vi "nanocal -- nuclear schottky fit V8.vi"() -> ()   [LabVIEW 2021] (continued)
  out "color data":cluster{"Array":dbl[], "Array":dbl[]}[](array[cluster])=[{"Array"=[0.12, 0.148, 0.179, 0.197, 0.249, 0.3, 0.36, 0.43, 0.512, 0.61, 0.81, 1.1, 1.8, 3.0, 5.7], "Array"=[0.375235391174, 0.267189614091, 0.199306617611, 0.169435500052, 0.10023219366, 0.068889386962, 0.050855621628, 0.038379394547, 0.030757711173, 0.024472356387, 0.019125590894, 0.016340595254, 0.01263439258, 0.019026086981, 0.019858524497]}, {"Array"=[0.12, 0.148, 0.179, 0.197, 0.249, 0.3, 0.36, 0.43, 0.512, 0.61, 0.81, 1.1, 1.8, 3.0, 5.7], "Array"=[0.100390183494, 0.086925369127, 0.070107577087, 0.06552222252, 0.0499817149, 0.042189760597, 0.035114064267, 0.030049345911, 0.024931554661, 0.022407083343, 0.016432131318, 0.01691523202, 0.012311180561, 0.018297259133, 0.012821278093]}, {"Array"=[0.12, 0.148, 0.179, 0.197, 0.249, 0.3, 0.36, 0.43, 0.512, 0.61, 0.81, 1.1, 1.8, 3.0, 5.7], "Array"=[0.059883674441, 0.044416499058, 0.034354681127, 0.031885966152, 0.026964705596, 0.023837806105, 0.021745076003, 0.020197203084, 0.019059366283, 0.017600386438, 0.016139955363, 0.015114072822, 0.011880374999, 0.007367031681, 0.004631070276]}, {"Array"=[0.12, 0.148, 0.179, 0.197, 0.249, 0.3, 0.36, 0.43, 0.512, 0.61, 0.81, 1.1, 1.8, 3.0, 5.7], "Array"=[0.583268417564, 0.254096954422, 0.115326183519, 0.085736532349, 0.034498560244, 0.017176281362, 0.009940720882, 0.005279271749, 0.002804912424, 0.001730254025, 0.000695948251, 0.000265648688, 6.6834392e-05, 1.2328467e-05, 1.621029e-06]}, {"Array"=[0.12, 0.148, 0.179, 0.197, 0.249, 0.3, 0.36, 0.43, 0.512, 0.61, 0.81, 1.1, 1.8, 3.0, 5.7], "Array"=[0.00101538821, 0.000963914391, 0.001029913549, 0.00108551185, 0.001422553924, 0.001657645209, 0.002035754152, 0.002296433055, 0.00240095569, 0.003444856237, 0.003787605771, 0.003610389555, 0.00409358538, 0.005085235141, 0.003887972994]}, {"Array"=[0.12, 0.148, 0.179, 0.197, 0.249, 0.3, 0.36, 0.43, 0.512, 0.61, 0.81, 1.1, 1.8, 3.0, 5.7], "Array"=[4.51e-10, 6.59e-10, 9.06e-10, 1.071e-09, 1.37e-09, 1.746e-09, 2.124e-09, 2.676e-09, 3.344e-09, 3.989e-09, 5.582e-09, 7.797e-09, 1.3452e-08, 2.3922e-08, 5.8873e-08]}, {"Array"=[0.12, 0.148, 0.179, 0.197, 0.249, 0.3, 0.36, 0.43, 0.512, 0.61, 0.81, 1.1, 1.8, 3.0, 5.7], "Array"=[0.000375271363, 0.000162673595, 8.029081e-05, 5.7538627e-05, 9.1233173e-05, 7.1502532e-05, 5.116404e-05, 5.9898317e-05, 8.8127283e-05, 8.7154359e-05, 0.000129667374, 0.000367130935, 0.000860954265, 0.473735460179, 6.096146916988]}, {"Array"=[0.12, 0.148, 0.179, 0.197, 0.249, 0.3, 0.36, 0.43, 0.512, 0.61, 0.81, 1.1, 1.8, 3.0, 5.7], "Array"=[0.000128650872, 3.6959811e-05, 1.3361577e-05, 8.322484e-06, 9.463067e-06, 5.082442e-06, 2.904884e-06, 2.370734e-06, 2.53316e-06, 1.846195e-06, 1.793381e-06, 1.790268e-06, 1.598192e-06, 0.000298320672, 0.000788360465]}, {"Array"=[0.12, 0.148, 0.179, 0.197, 0.249, 0.3, 0.36, 0.43, 0.512, 0.61, 0.81, 1.1, 1.8, 3.0, 5.7], "Array"=[0.00159846382, 0.000362772077, 0.000100930245, 5.7382706e-05, 4.5871847e-05, 2.0526312e-05, 9.775078e-06, 6.802565e-06, 6.068263e-06, 3.983538e-06, 2.982571e-06, 3.209434e-06, 2.482039e-06, 0.226260580227, 2.944305334628]}, {"Array"=[0.12, 0.148, 0.179, 0.197, 0.249, 0.3, 0.36, 0.43, 0.512, 0.61, 0.81, 1.1, 1.8, 3.0, 5.7], "Array"=[0.003738128067, 0.00187141679, 0.001145251526, 0.000878154381, 0.00182533099, 0.001694784024, 0.001457081108, 0.001993331815, 0.003534768852, 0.003889589636, 0.007891086787, 0.021704161954, 0.06993271366, 0.0, 0.0]}, {"Array"=[0.12, 0.148, 0.179, 0.197, 0.249, 0.3, 0.36, 0.43, 0.512, 0.61, 0.81, 1.1, 1.8, 3.0, 5.7], "Array"=[0.002148346326, 0.000832118957, 0.000388930305, 0.000261007731, 0.000350942719, 0.000213209307, 0.000133588143, 0.000117379325, 0.00013290891, 0.000104895132, 0.000111114402, 0.000118450384, 0.000134523688, 0.0, 0.0]}, {"Array"=[0.12, 0.148, 0.179, 0.197, 0.249, 0.3, 0.36, 0.43, 0.512, 0.61, 0.81, 1.1, 1.8, 3.0, 5.7], "Array"=[0.002740528669, 0.00142769156, 0.000875171988, 0.000669291195, 0.001329674256, 0.00119503816, 0.000983336979, 0.001288542279, 0.002163441144, 0.002302284973, 0.004285622428, 0.012081499151, 0.037137152263, 0.0, 0.0]}, {"Array"=[0.12, 0.148, 0.179, 0.197, 0.249, 0.3, 0.36, 0.43, 0.512, 0.61, 0.81, 1.1, 1.8, 3.0, 5.7], "Array"=[0.004856405038, 0.00339935422, 0.002396778835, 0.002148162128, 0.001574610259, 0.001314390211, 0.001126696289, 0.000994558397, 0.000873567124, 0.000814716505, 0.00067871105, 0.000664500257, 0.000525383024, 0.0, 0.0]}, {"Array"=[0.12, 0.148, 0.179, 0.197, 0.249, 0.3, 0.36, 0.43, 0.512, 0.61, 0.81, 1.1, 1.8, 3.0, 5.7], "Array"=[0.000120937865, 6.5769536e-05, 3.6147224e-05, 2.8270387e-05, 1.5357324e-05, 8.848315e-06, 6.319561e-06, 4.045439e-06, 2.751674e-06, 1.970451e-06, 1.210723e-06, 3.99152e-07, 1.29432e-07, 0.0, 0.0]}, {"Array"=[0.12, 0.148, 0.179, 0.197, 0.249, 0.3, 0.36, 0.43, 0.512, 0.61, 0.81, 1.1, 1.8, 3.0, 5.7], "Array"=[0.036262763887, 0.013360978569, 0.005461206603, 0.003934877132, 0.001506729222, 0.000735278812, 0.000424808302, 0.000225535524, 0.000120705086, 7.4828897e-05, 3.0773e-05, 1.1616244e-05, 2.96677e-06, 0.0, 0.0]}, {"Array"=[0.12, 0.148, 0.179, 0.197, 0.249, 0.3, 0.36, 0.43, 0.512, 0.61, 0.81, 1.1, 1.8, 3.0, 5.7], "Array"=[0.04837529795, 0.039106583663, 0.034187158287, 0.032785245148, 0.03150372616, 0.031154246719, 0.032086752475, 0.033097505686, 0.03503861415, 0.036359774839, 0.041303896436, 0.039284134925, 0.042675275628, 0.0, 0.0]}, {"Array"=[0.12, 0.148, 0.179, 0.197, 0.249, 0.3, 0.36, 0.43, 0.512, 0.61, 0.81, 1.1, 1.8, 3.0, 5.7], "Array"=[0.0020195465, 0.001480745607, 0.001052177546, 0.000886609066, 0.000569534267, 0.000371188322, 0.00029062032, 0.000200297015, 0.000144373831, 0.000111954983, 7.5013998e-05, 2.6409322e-05, 1.0894575e-05, 0.0, 0.0]}, {"Array"=[0.12, 0.148, 0.179, 0.197, 0.249, 0.3, 0.36, 0.43, 0.512, 0.61, 0.81, 1.1, 1.8, 3.0, 5.7], "Array"=[0.062171656813, 0.05258220666, 0.047354437967, 0.045894988103, 0.043675133431, 0.042807799707, 0.042734154502, 0.042720953668, 0.043033459724, 0.043247347257, 0.044217367932, 0.043727840988, 0.044389870063, 0.0, 0.0]}, {"Array"=[0.12, 0.148, 0.179, 0.197, 0.249, 0.3, 0.36, 0.43, 0.512, 0.61, 0.81, 1.1, 1.8, 3.0, 5.7], "Array"=[0.0, 0.0, 0.0, 0.0, 0.0, 0.0, 0.0, 0.0, 0.0, 0.0, 0.0, 0.0, 0.0, -126530.61224489775, -53061.22448979574]}, {"Array"=[0.12, 0.148, 0.179, 0.197, 0.249, 0.3, 0.36, 0.43, 0.512, 0.61, 0.81, 1.1, 1.8, 3.0, 5.7], "Array"=[0.0, 0.0, 0.0, 0.0, 0.0, 0.0, 0.0, 0.0, 0.0, 0.0, 0.0, 0.0, 0.0, 0.0, 0.0]}, {"Array"=[0.12, 0.148, 0.179, 0.197, 0.249, 0.3, 0.36, 0.43, 0.512, 0.61, 0.81, 1.1, 1.8, 3.0, 5.7], "Array"=[0.0, 0.0, 0.0, 0.0, 0.0, 0.0, 0.0, 0.0, 0.0, 0.0, 0.0, 0.0, 0.0, 0.0, 0.0]}]
  out "R(ω) fit out":cdb[](array[numeric])
  in  "parameter map":map{T1, dbl}(c390)={enum."ζ"=0.068889386962, enum."τ1"=0.042189760597, enum."τS"=0.023837806105, enum."τN"=0.017176281362, enum."τC"=0.001657645209, enum."κ0"=1.746e-09}
  out "filesnames lookup":map{i32, string}(c390)={0="IDS0158_210310_RAW_cal__sam_", 1="IDS0183_210310_RAW_cal__sam_", 2="IDS0311_210901_RAW_cal__sam_", 3="IDS0359_210907_RAW_cal__sam_", 4="IDS0412_220525_RAW_cal__sam_", 5="IDS0431_220527_RAW_cal__sam_", 6="IDS0442_220528_RAW_cal__sam_", 7="IDS0464_220530_RAW_cal__sam_", 8="IDS0486_220602_RAW_cal__sam_", 9="IDS0495_220602_RAW_cal__sam_", 10="IDS0510_220603_RAW_cal__sam_", 11="IDS0526_220605_RAW_cal__sam_", 12="IDS0544_220606_RAW_cal__sam_", 13="IDS0561_220607_RAW_cal__sam_", 14="IDS0581_220608_RAW_cal__sam_", 15="IDS0598_220609_RAW_cal__sam_", 16="IDS0627_220611_RAW_cal__sam_", 17="IDS0643_220612_RAW_cal__sam_", 18="IDS0336_210904_RAW_cal__sam_", 19="IDS0346_210904_RAW_cal__sam_", 20="IDS0378_210909_RAW_cal__sam_", 21="IDS0300_210427_RAW_cal__sam_", 22="IDS0184_210310_RAW_cal__sam_", 23="IDS0210_210310_RAW_cal__sam_", 24="IDS0379_210909_RAW_cal__sam_", 25="IDS0159_210310_RAW_cal__sam_", 26="IDS0360_210907_RAW_cal__sam_", 27="IDS0411_220525_RAW_cal__sam_", 28="IDS0427_220526_RAW_cal__sam_", 29="IDS0443_220528_RAW_cal__sam_", 30="IDS0463_220530_RAW_cal__sam_", 31="IDS0487_220602_RAW_cal__sam_", 32="IDS0496_220602_RAW_cal__sam_", 33="IDS0509_220603_RAW_cal__sam_", 34="IDS0525_220605_RAW_cal__sam_", 35="IDS0543_220606_RAW_cal__sam_", 36="IDS0560_220607_RAW_cal__sam_", 37="IDS0580_220608_RAW_cal__sam_", 38="IDS0597_220608_RAW_cal__sam_", 39="IDS0626_220611_RAW_cal__sam_", 40="IDS0642_220612_RAW_cal__sam_", 41="IDS0310_210901_RAW_cal__sam_", 42="IDS0337_210904_RAW_cal__sam_", 43="IDS0347_210906_RAW_cal__sam_", 44="IDS0305_210831_RAW_cal__sam_", 45="IDS0361_210908_RAW_cal__sam_", 46="IDS0380_210909_RAW_cal__sam_", 47="IDS0304_210831_RAW_cal__sam_", 48="IDS0312_210901_RAW_cal__sam_", 49="IDS0338_210904_RAW_cal__sam_", 50="IDS0410_220525_RAW_cal__sam_", 51="IDS0432_220527_RAW_cal__sam_", 52="IDS0444_220528_RAW_cal__sam_", 53="IDS0462_220530_RAW_cal__sam_", 54="IDS0485_220601_RAW_cal__sam_", 55="IDS0497_220603_RAW_cal__sam_", 56="IDS0511_220604_RAW_cal__sam_", 57="IDS0524_220605_RAW_cal__sam_", 58="IDS0542_220606_RAW_cal__sam_", 59="IDS0559_220607_RAW_cal__sam_", 60="IDS0579_220608_RAW_cal__sam_", 61="IDS0596_220608_RAW_cal__sam_", 62="IDS0625_220611_RAW_cal__sam_", 63="IDS0641_220612_RAW_cal__sam_", 64="IDS0348_210906_RAW_cal__sam_", 65="IDS0181_210310_RAW_cal__sam_", 66="IDS0160_210310_RAW_cal__sam_", 67="IDS0424_220526_RAW_cal__sam_", 68="IDS0185_210310_RAW_cal__sam_", 69="IDS0208_210310_RAW_cal__sam_", 70="IDS0209_210310_RAW_cal__sam_", 71="IDS0211_210310_RAW_cal__sam_", 72="IDS0212_210310_RAW_cal__sam_", 73="IDS0213_210310_RAW_cal__sam_", 74="IDS0214_210310_RAW_cal__sam_", 75="IDS0215_210310_RAW_cal__sam_", 76="IDS0216_210310_RAW_cal__sam_", 77="IDS0217_210310_RAW_cal__sam_", 78="IDS0330_210901_RAW_cal__sam_", 79="IDS0331_210901_RAW_cal__sam_", 80="IDS0335_210904_RAW_cal__sam_", 81="IDS0362_210908_RAW_cal__sam_", 82="IDS0377_210909_RAW_cal__sam_", 83="IDS0161_210310_RAW_cal__sam_", 84="IDS0303_210831_RAW_cal__sam_", 85="IDS0313_210901_RAW_cal__sam_", 86="IDS0349_210906_RAW_cal__sam_", 87="IDS0407_220525_RAW_cal__sam_", 88="IDS0441_220527_RAW_cal__sam_", 89="IDS0458_220529_RAW_cal__sam_", 90="IDS0477_220601_RAW_cal__sam_", 91="IDS0493_220602_RAW_cal__sam_", 92="IDS0508_220603_RAW_cal__sam_", 93="IDS0523_220604_RAW_cal__sam_", 94="IDS0540_220605_RAW_cal__sam_", 95="IDS0562_220607_RAW_cal__sam_", 96="IDS0578_220608_RAW_cal__sam_", 97="IDS0595_220608_RAW_cal__sam_", 98="IDS0624_220611_RAW_cal__sam_", 99="IDS0640_220612_RAW_cal__sam_", 100="IDS0186_210310_RAW_cal__sam_", 101="IDS0162_210310_RAW_cal__sam_", 102="IDS0302_210831_RAW_cal__sam_", 103="IDS0363_210908_RAW_cal__sam_", 104="IDS0381_210909_RAW_cal__sam_", 105="IDS0408_220525_RAW_cal__sam_", 106="IDS0425_220526_RAW_cal__sam_", 107="IDS0445_220528_RAW_cal__sam_", 108="IDS0459_220529_RAW_cal__sam_", 109="IDS0478_220601_RAW_cal__sam_", 110="IDS0494_220602_RAW_cal__sam_", 111="IDS0512_220604_RAW_cal__sam_", 112="IDS0527_220605_RAW_cal__sam_", 113="IDS0541_220605_RAW_cal__sam_", 114="IDS0563_220607_RAW_cal__sam_", 115="IDS0582_220608_RAW_cal__sam_", 116="IDS0599_220609_RAW_cal__sam_", 117="IDS0628_220611_RAW_cal__sam_", 118="IDS0644_220612_RAW_cal__sam_", 119="IDS0314_210901_RAW_cal__sam_", 120="IDS0339_210904_RAW_cal__sam_", 121="IDS0350_210906_RAW_cal__sam_", 122="IDS0163_210310_RAW_cal__sam_", 123="IDS0187_210310_RAW_cal__sam_", 124="IDS0301_210831_RAW_cal__sam_", 125="IDS0315_210901_RAW_cal__sam_", 126="IDS0382_210909_RAW_cal__sam_", 127="IDS0409_220525_RAW_cal__sam_", 128="IDS0426_220526_RAW_cal__sam_", 129="IDS0446_220528_RAW_cal__sam_", 130="IDS0460_220529_RAW_cal__sam_", 131="IDS0479_220601_RAW_cal__sam_", 132="IDS0498_220603_RAW_cal__sam_", 133="IDS0513_220604_RAW_cal__sam_", 134="IDS0528_220605_RAW_cal__sam_", 135="IDS0545_220606_RAW_cal__sam_", 136="IDS0564_220607_RAW_cal__sam_", 137="IDS0583_220608_RAW_cal__sam_", 138="IDS0629_220611_RAW_cal__sam_", 139="IDS0645_220612_RAW_cal__sam_", 140="IDS0656_220614_RAW_cal__sam_", 141="IDS0364_210908_RAW_cal__sam_", 142="IDS0340_210904_RAW_cal__sam_", 143="IDS0351_210906_RAW_cal__sam_", 144="IDS0164_210310_RAW_cal__sam_", 145="IDS0188_210310_RAW_cal__sam_", 146="IDS0299_210427_RAW_cal__sam_", 147="IDS0316_210901_RAW_cal__sam_", 148="IDS0341_210904_RAW_cal__sam_", 149="IDS0352_210906_RAW_cal__sam_", 150="IDS0365_210908_RAW_cal__sam_", 151="IDS0383_210910_RAW_cal__sam_", 152="IDS0413_220525_RAW_cal__sam_", 153="IDS0428_220526_RAW_cal__sam_", 154="IDS0447_220528_RAW_cal__sam_", 155="IDS0461_220529_RAW_cal__sam_", 156="IDS0480_220601_RAW_cal__sam_", 157="IDS0499_220603_RAW_cal__sam_", 158="IDS0514_220604_RAW_cal__sam_", 159="IDS0529_220605_RAW_cal__sam_", 160="IDS0546_220606_RAW_cal__sam_", 161="IDS0565_220607_RAW_cal__sam_", 162="IDS0584_220608_RAW_cal__sam_", 163="IDS0601_220609_RAW_cal__sam_", 164="IDS0630_220611_RAW_cal__sam_", 165="IDS0646_220612_RAW_cal__sam_", 166="IDS0429_220526_RAW_cal__sam_", 167="IDS0448_220528_RAW_cal__sam_", 168="IDS0481_220601_RAW_cal__sam_", 169="IDS0500_220603_RAW_cal__sam_", 170="IDS0530_220605_RAW_cal__sam_", 171="IDS0547_220606_RAW_cal__sam_", 172="IDS0566_220607_RAW_cal__sam_", 173="IDS0585_220608_RAW_cal__sam_", 174="IDS0602_220609_RAW_cal__sam_", 175="IDS0631_220611_RAW_cal__sam_", 176="IDS0647_220612_RAW_cal__sam_", 177="IDS0165_210310_RAW_cal__sam_", 178="IDS0189_210310_RAW_cal__sam_", 179="IDS0298_210427_RAW_cal__sam_", 180="IDS0317_210901_RAW_cal__sam_", 181="IDS0366_210908_RAW_cal__sam_", 182="IDS0384_210910_RAW_cal__sam_", 183="IDS0414_220525_RAW_cal__sam_", 184="IDS0465_220530_RAW_cal__sam_", 185="IDS0515_220604_RAW_cal__sam_", 186="IDS0342_210904_RAW_cal__sam_", 187="IDS0353_210906_RAW_cal__sam_", 188="IDS0190_210310_RAW_cal__sam_", 189="IDS0166_210310_RAW_cal__sam_", 190="IDS0430_220526_RAW_cal__sam_", 191="IDS0449_220528_RAW_cal__sam_", 192="IDS0482_220601_RAW_cal__sam_", 193="IDS0501_220603_RAW_cal__sam_", 194="IDS0516_220604_RAW_cal__sam_", 195="IDS0531_220605_RAW_cal__sam_", 196="IDS0548_220606_RAW_cal__sam_", 197="IDS0567_220607_RAW_cal__sam_", 198="IDS0586_220608_RAW_cal__sam_", 199="IDS0603_220609_RAW_cal__sam_", 200="IDS0632_220611_RAW_cal__sam_", 201="IDS0648_220613_RAW_cal__sam_", 202="IDS0297_210427_RAW_cal__sam_", 203="IDS0318_210901_RAW_cal__sam_", 204="IDS0343_210904_RAW_cal__sam_", 205="IDS0354_210906_RAW_cal__sam_", 206="IDS0367_210908_RAW_cal__sam_", 207="IDS0385_210910_RAW_cal__sam_", 208="IDS0415_220525_RAW_cal__sam_", 209="IDS0466_220530_RAW_cal__sam_", 210="IDS0191_210310_RAW_cal__sam_", 211="IDS0167_210310_RAW_cal__sam_", 212="IDS0296_210427_RAW_cal__sam_", 213="IDS0319_210901_RAW_cal__sam_", 214="IDS0344_210904_RAW_cal__sam_", 215="IDS0433_220527_RAW_cal__sam_", 216="IDS0450_220528_RAW_cal__sam_", 217="IDS0467_220530_RAW_cal__sam_", 218="IDS0483_220601_RAW_cal__sam_", 219="IDS0502_220603_RAW_cal__sam_", 220="IDS0517_220604_RAW_cal__sam_", 221="IDS0532_220605_RAW_cal__sam_", 222="IDS0549_220606_RAW_cal__ref_", 223="IDS0568_220607_RAW_cal__sam_", 224="IDS0587_220608_RAW_cal__sam_", 225="IDS0604_220609_RAW_cal__sam_", 226="IDS0618_220610_RAW_cal__sam_", 227="IDS0633_220611_RAW_cal__sam_", 228="IDS0649_220613_RAW_cal__sam_", 229="IDS0368_210908_RAW_cal__sam_", 230="IDS0386_210910_RAW_cal__sam_", 231="IDS0416_220525_RAW_cal__sam_", 232="IDS0220_210310_RAW_cal__sam_", 233="IDS0168_210310_RAW_cal__sam_", 234="IDS0192_210310_RAW_cal__sam_", 235="IDS0434_220527_RAW_cal__sam_", 236="IDS0451_220528_RAW_cal__sam_", 237="IDS0468_220530_RAW_cal__sam_", 238="IDS0484_220601_RAW_cal__sam_", 239="IDS0503_220603_RAW_cal__sam_", 240="IDS0518_220604_RAW_cal__sam_", 241="IDS0533_220605_RAW_cal__sam_", 242="IDS0550_220606_RAW_cal__sam_", 243="IDS0569_220607_RAW_cal__sam_", 244="IDS0588_220608_RAW_cal__sam_", 245="IDS0605_220609_RAW_cal__sam_", 246="IDS0612_220610_RAW_cal__sam_", 247="IDS0634_220612_RAW_cal__sam_", 248="IDS0650_220613_RAW_cal__sam_", 249="IDS0295_210427_RAW_cal__sam_", 250="IDS0320_210901_RAW_cal__sam_", 251="IDS0355_210906_RAW_cal__sam_", 252="IDS0369_210908_RAW_cal__sam_", 253="IDS0387_210910_RAW_cal__sam_", 254="IDS0417_220525_RAW_cal__sam_", 255="IDS0219_210310_RAW_cal__sam_", 256="IDS0193_210310_RAW_cal__sam_", 257="IDS0606_220609_RAW_cal__sam_", 258="IDS0169_210310_RAW_cal__sam_", 259="IDS0418_220525_RAW_cal__sam_", 260="IDS0435_220527_RAW_cal__sam_", 261="IDS0452_220528_RAW_cal__sam_", 262="IDS0469_220530_RAW_cal__sam_", 263="IDS0488_220602_RAW_cal__sam_", 264="IDS0504_220603_RAW_cal__sam_", 265="IDS0519_220604_RAW_cal__sam_", 266="IDS0534_220605_RAW_cal__sam_", 267="IDS0551_220606_RAW_cal__sam_", 268="IDS0570_220607_RAW_cal__sam_", 269="IDS0589_220608_RAW_cal__sam_", 270="IDS0613_220610_RAW_cal__sam_", 271="IDS0619_220610_RAW_cal__sam_", 272="IDS0635_220612_RAW_cal__sam_", 273="IDS0651_220613_RAW_cal__sam_", 274="IDS0294_210427_RAW_cal__sam_", 275="IDS0321_210901_RAW_cal__sam_", 276="IDS0370_210908_RAW_cal__sam_", 277="IDS0388_210910_RAW_cal__sam_", 278="IDS0391_210910_RAW_cal__sam_", 279="IDS0439_220527_RAW_cal__sam_", 280="IDS0395_210910_RAW_cal__sam_", 281="IDS0392_210910_RAW_cal__sam_", 282="IDS0556_220606_RAW_cal__sam_", 283="IDS0389_210910_RAW_cal__sam_", 284="IDS0218_210310_RAW_cal__sam_", 285="IDS0590_220608_RAW_cal__sam_", 286="IDS0607_220609_RAW_cal__sam_", 287="IDS0453_220529_RAW_cal__sam_", 288="IDS0535_220605_RAW_cal__sam_", 289="IDS0170_210310_RAW_cal__sam_", 290="IDS0194_210310_RAW_cal__sam_", 291="IDS0293_210427_RAW_cal__sam_", 292="IDS0322_210901_RAW_cal__sam_", 293="IDS0371_210908_RAW_cal__sam_", 294="IDS0390_210910_RAW_cal__sam_", 295="IDS0419_220525_RAW_cal__sam_", 296="IDS0436_220527_RAW_cal__sam_", 297="IDS0454_220529_RAW_cal__sam_", 298="IDS0470_220530_RAW_cal__sam_", 299="IDS0489_220602_RAW_cal__sam_", 300="IDS0505_220603_RAW_cal__sam_", 301="IDS0520_220604_RAW_cal__sam_", 302="IDS0536_220605_RAW_cal__sam_", 303="IDS0552_220606_RAW_cal__sam_", 304="IDS0571_220607_RAW_cal__sam_", 305="IDS0608_220610_RAW_cal__sam_", 306="IDS0614_220610_RAW_cal__sam_", 307="IDS0620_220610_RAW_cal__sam_", 308="IDS0636_220612_RAW_cal__sam_", 309="IDS0652_220613_RAW_cal__sam_", 310="IDS0420_220525_RAW_cal__sam_", 311="IDS0421_220525_RAW_cal__sam_", 312="IDS0471_220530_RAW_cal__sam_", 313="IDS0553_220606_RAW_cal__sam_", 314="IDS0572_220607_RAW_cal__sam_", 315="IDS0591_220608_RAW_cal__sam_", 316="IDS0195_210310_RAW_cal__sam_", 317="IDS0472_220530_RAW_cal__sam_", 318="IDS0171_210310_RAW_cal__sam_", 319="IDS0306_210831_RAW_cal__sam_", 320="IDS0323_210901_RAW_cal__sam_", 321="IDS0422_220525_RAW_cal__sam_", 322="IDS0437_220527_RAW_cal__sam_", 323="IDS0455_220529_RAW_cal__sam_", 324="IDS0490_220602_RAW_cal__sam_", 325="IDS0506_220603_RAW_cal__sam_", 326="IDS0521_220604_RAW_cal__sam_", 327="IDS0537_220605_RAW_cal__sam_", 328="IDS0554_220606_RAW_cal__sam_", 329="IDS0573_220607_RAW_cal__sam_", 330="IDS0592_220608_RAW_cal__sam_", 331="IDS0609_220610_RAW_cal__sam_", 332="IDS0615_220610_RAW_cal__sam_", 333="IDS0621_220610_RAW_cal__sam_", 334="IDS0637_220612_RAW_cal__sam_", 335="IDS0653_220613_RAW_cal__sam_", 336="IDS0372_210908_RAW_cal__sam_", 337="IDS0393_210910_RAW_cal__sam_", 338="IDS0172_210310_RAW_cal__sam_", 339="IDS0196_210310_RAW_cal__sam_", 340="IDS0324_210901_RAW_cal__sam_", 341="IDS0438_220527_RAW_cal__sam_", 342="IDS0456_220529_RAW_cal__sam_", 343="IDS0473_220531_RAW_cal__sam_", 344="IDS0491_220602_RAW_cal__sam_", 345="IDS0538_220605_RAW_cal__sam_", 346="IDS0555_220606_RAW_cal__sam_", 347="IDS0574_220607_RAW_cal__sam_", 348="IDS0593_220608_RAW_cal__sam_", 349="IDS0610_220610_RAW_cal__sam_", 350="IDS0616_220610_RAW_cal__sam_", 351="IDS0622_220610_RAW_cal__sam_", 352="IDS0638_220612_RAW_cal__sam_", 353="IDS0654_220613_RAW_cal__sam_", 354="IDS0373_210908_RAW_cal__sam_", 355="IDS0394_210910_RAW_cal__sam_"}
  out "constrained filename lookup":map{i32, string}(c390)={0="IDS0183_210310_RAW_cal__ref_", 1="IDS0184_210310_RAW_cal__ref_", 2="IDS0181_210310_RAW_cal__ref_", 3="IDS0185_210310_RAW_cal__ref_", 4="IDS0186_210310_RAW_cal__ref_", 5="IDS0187_210310_RAW_cal__ref_", 6="IDS0188_210310_RAW_cal__ref_", 7="IDS0189_210310_RAW_cal__ref_", 8="IDS0190_210310_RAW_cal__ref_", 9="IDS0191_210310_RAW_cal__ref_", 10="IDS0192_210310_RAW_cal__ref_", 11="IDS0193_210310_RAW_cal__ref_", 12="IDS0194_210310_RAW_cal__ref_", 13="IDS0195_210310_RAW_cal__ref_", 14="IDS0196_210310_RAW_cal__ref_"}
  out "mathematica thing":map{string, map{T1, dbl}}(c390)
  out "temps&degs":map{string, map{T1, dbl}}(c390)
  out "all short filenames":map{string, string}(c390)
  out "all full filenames":map{string, path}(c390)
  out "data file parameters map":map{T1, T13}(c390)={enum."T (K)"=enum."get T", enum."B (T)"=enum."get B", enum."θ (deg)"=enum."get deg", enum."set of (B|T)"=enum."get setof"}
  out "side map to NUM":map{T9, i32}(c390)={enum."sam"=8000, enum."ref"=4000}
  out "side map to STR":map{T9, string}(c390)={enum."sam"="_sam_", enum."ref"="_ref_"}
  out "side map from NUM":map{i32, T9}(c390)={4000=enum."ref", 8000=enum."sam"}
  in  "reverse cursor index map":map{i32, T1}(c390)={0=enum."ζ", 1=enum."τ1", 2=enum."τS", 3=enum."τN", 4=enum."τC", 5=enum."κ0", 6=enum."m1", 7=enum."m2", 8=enum."m3"}
  out "state of all selectors":map{T1, map{bool, dbl}}(c390)={enum."T (K)"={TRUE=0.122}, enum."B (T)"={FALSE=12.0}, enum."θ (deg)"={FALSE=90.0}, enum."side (S|R)"={FALSE=4000.0}, enum."set of (B|T)"={TRUE=1.0}}
  out "state of all selectors string":string="__12T__90deg__4000side_"
  out "new selector names":map{T1, map{T14, string}}(c390)={enum."ζ"={enum."name"="ζ", enum."nameL"="zeta", enum."units"="sec", enum."prec"="%_4p"}, enum."τ1"={enum."name"="τ1", enum."nameL"="tau1", enum."units"="sec", enum."prec"="%_4p"}, enum."τS"={enum."name"="τS", enum."nameL"="tauS", enum."units"="sec", enum."prec"="%_4p"}, enum."τN"={enum."name"="τN", enum."nameL"="tauN", enum."units"="sec", enum."prec"="%_4p"}, enum."τC"={enum."name"="τC", enum."nameL"="tauC", enum."units"="sec", enum."prec"="%_4p"}, enum."κ0"={enum."name"="κ0", enum."nameL"="kappa0", enum."units"="WperK", enum."prec"="%_5p"}, enum."T (K)"={enum."name"="T", enum."nameL"="T", enum."units"="K", enum."prec"="%_4p"}, enum."B (T)"={enum."name"="B", enum."nameL"="B", enum."units"="T", enum."prec"="%_2p"}, enum."θ (deg)"={enum."name"="θ", enum."nameL"="theta", enum."units"="deg", enum."prec"="%_2p"}, enum."side (S|R)"={enum."name"="side", enum."nameL"="side", enum."units"="side", enum."prec"="%d"}, enum."Re(offset)"={enum."name"="Reoffset", enum."nameL"="Reoffset", enum."units"="au", enum."prec"="%_4p"}, enum."Im(offset)"={enum."name"="Imoffset", enum."nameL"="Imoffset", enum."units"="au", enum."prec"="%_4p"}, enum."στ1"={enum."name"="στ1", enum."nameL"="sigmatau1", enum."units"="sec", enum."prec"="%_4p"}, enum."στS"={enum."name"="στS", enum."nameL"="sigmatauS", enum."units"="sec", enum."prec"="%_4p"}, enum."στN"={enum."name"="στN", enum."nameL"="sigmatauN", enum."units"="sec", enum."prec"="%_4p"}, enum."τ11"={enum."name"="τ11", enum."nameL"="tau11", enum."units"="sec", enum."prec"="%_4p"}, enum."τ12"={enum."name"="τ12", enum."nameL"="tau12", enum."units"="sec", enum."prec"="%_4p"}, enum."τ22"={enum."name"="τ22", enum."nameL"="tau22", enum."units"="sec", enum."prec"="%_4p"}, enum."τN1"={enum."name"="τN1", enum."nameL"="tauN1", enum."units"="sec", enum."prec"="%_4p"}, enum."τN2"={enum."name"="τN2", enum."nameL"="tauN2", enum."units"="sec", enum."prec"="%_4p"}, enum."σηlogτ1"={enum."name"="σηlogτ1", enum."nameL"="sigmaetalogtau1", enum."units"="au", enum."prec"="%_4p"}, enum."σηlogτS"={enum."name"="σηlogτS", enum."nameL"="sigmaetalogtauS", enum."units"="au", enum."prec"="%_4p"}, enum."σηlogτN"={enum."name"="σηlogτN", enum."nameL"="sigmaetalogtauN", enum."units"="au", enum."prec"="%_4p"}, enum."σlogτ1"={enum."name"="σlogτ1", enum."nameL"="sigmalogtau1", enum."units"="au", enum."prec"="%_4p"}, enum."σlogτS"={enum."name"="σlogτS", enum."nameL"="sigmalogtauS", enum."units"="au", enum."prec"="%_4p"}, enum."σlogτN"={enum."name"="σlogτN", enum."nameL"="sigmalogtauN", enum."units"="au", enum."prec"="%_4p"}, enum."σητ1"={enum."name"="σητ1", enum."nameL"="sigmaetatau1", enum."units"="sec", enum."prec"="%_4p"}, enum."σητS"={enum."name"="σητS", enum."nameL"="sigmaetatauS", enum."units"="sec", enum."prec"="%_4p"}, enum."σητN"={enum."name"="σητN", enum."nameL"="sigmaetatauN", enum."units"="sec", enum."prec"="%_4p"}, enum."noiseT"={enum."name"="noiseT", enum."nameL"="noiseT", enum."units"="au", enum."prec"="%_4p"}}
  in  "cursor index map":map{T1, i32}(c390)={enum."ζ"=0, enum."τ1"=1, enum."τS"=2, enum."τN"=3, enum."τC"=4, enum."κ0"=5, enum."m1"=6, enum."m2"=7, enum."m3"=8}
  in  "plotme waves":map{string, dbl[]}(c390)={"T     tauC     zeta"=array[558 elements]}
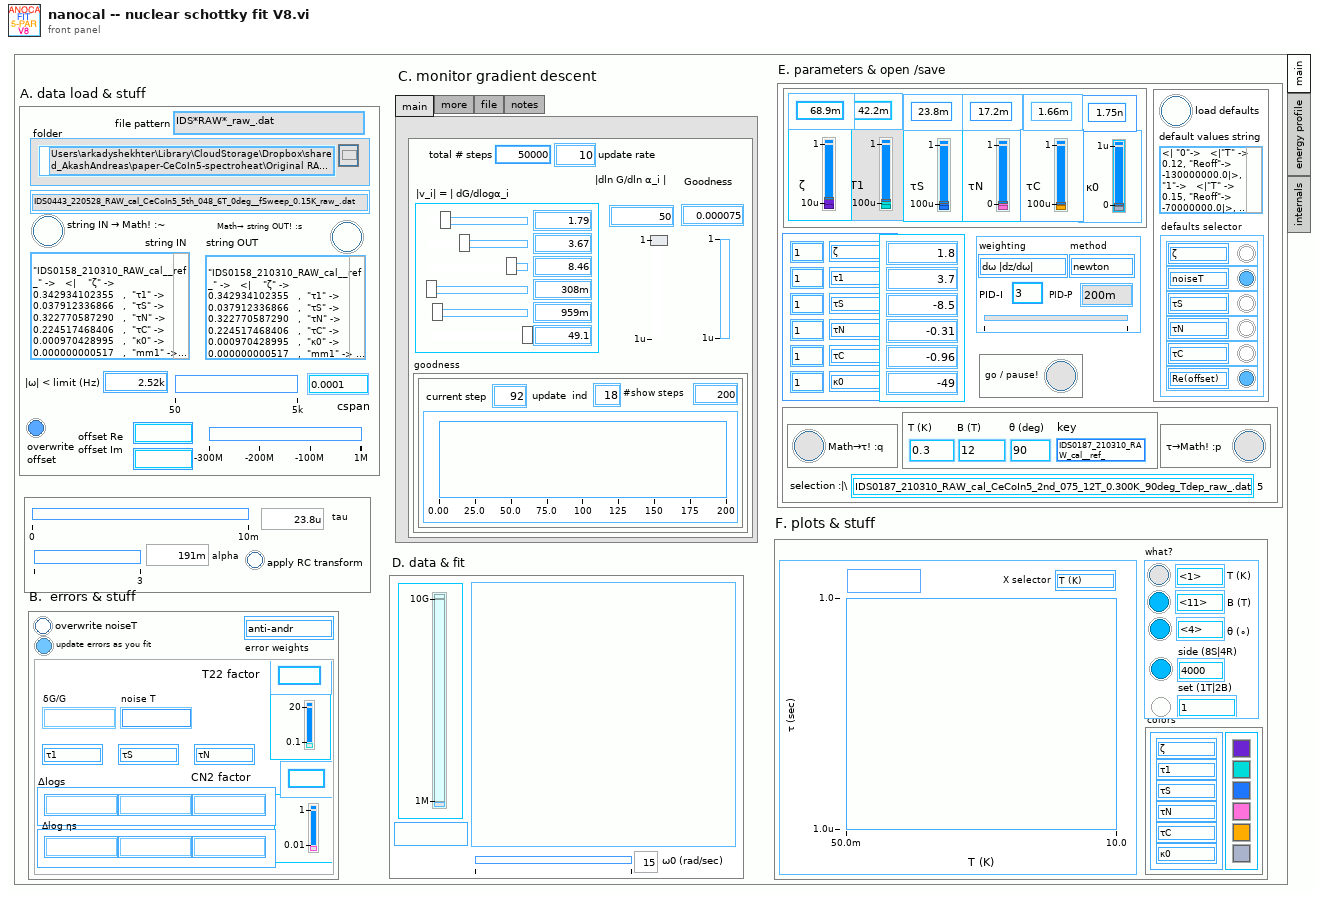
[diagram p1: front panel]
types:
  T1 = typedef "3-lorentzian-parameters.ctl" = enum16{"ζ", "τ1", "τS", "τN", "τC", "κ0", "m1", "m2", "m3", "T (K)", "B (T)", "θ (deg)", "side (S|R)", "set of (B|T)", "Re(offset)", "Im(offset)", "στ1", "στ1-", "στ1+", "στS", "στS-", "στS+", "στN", "στN-", "στN+", "τ11", "τ12", "τ21", "τ22", "τN1", "τN2", "σηlogτ1", "σηlogτS", "σηlogτN", "σlogτ1", "σlogτS", "σlogτN", "σητ1", "σητS", "σητN", "noiseT"}
  T2 = typedef "nanocal -- gradient descent -- parameters.ctl" = cluster{"method":T3, "weighting":T4, "PID-P":dbl, "PID-I":i32}
  T3 = typedef "linear regression type.ctl" = enum16{"ignore", "gradient", "newton"}
  T4 = typedef "nanocal-goodness-weighting-strategy.ctl" = enum16{"dω", "dω √(|dz/dω|)", "dω |dz/dω|", "phase", "andreas", "sum", "anti-andr", "ark"}
  T5 = cluster{"Plost: sweep window":T1, "used default":bool}[]
  T6 = cluster{"ignore set of !":bool, "set (1T|2B)":i32, "ignore side !":bool, "side (8S|4R)":i64, "ignore θ !":bool, "ignore B !":bool, "T (K)":dbl, "ignore T !":bool, "θ (∘)":dbl, "B (T)":dbl, "lookup":cluster{"set of lookup":map{i32, dbl}, "all set of":set{dbl}, "T lookup":map{i32, dbl}, "θ lookup":map{i32, dbl}, "B lookup":map{i32, dbl}, "all T's":set{dbl}, "all θ's":set{dbl}, "all B's":set{dbl}, "all sides":set{dbl}, "side lookup":map{i32, dbl}}}
  T7 = typedef "nanocal_data_read_format.ctl" = enum16{"as is", "add - ω", "full rydh", "raw nanocal"}
  T8 = typedef "filename-pattern.ctl" = cluster{"prefix":string, "group":string}
  T9 = typedef "nanocal_side_selector.ctl" = enum16{"sam", "ref"}
  T10 = typedef "3D curvature triplet control -- V2.ctl" = cluster{"one":T1, "two":T1, "sigmaone":T1, "sigmatwo":T1, "three":T1, "sigmathree":T1, "pars & errors":map{T1, dbl}, "T22 factor":dbl, "CN2 factor":dbl, "δG/G":dbl, "noise T":dbl, "Δlogs":dbl[], "Δlog ηs":dbl[]}
  T11 = typedef "show-win- control.ctl" = cluster{"cen (Hz)":dbl, "win (Hz)":dbl, "left (Hz)":dbl, "right (Hz)":dbl}
  T12 = typedef "cursor winow.ctl" = cluster{"left":dbl, "right ":dbl, "center":dbl, "window":dbl, "cursors":i32[], "relative":i32, "absolute":i32, "fixed vertical offset":dbl, "vertical offset":dbl, "skew":dbl, "default window frac":dbl, "kind":enum16{"symmetric", "skewed", "fancy"}, "skew.left":dbl, "skew.right":dbl, "Plot ref":refnum<vi>, "wing order":enum16{"forw", "back"}}
  T13 = typedef "filename-action.ctl" = enum16{"rewrite", "parse", "force pattern", "uniquenum", "get T", "get B", "get ind", "get deg", "get name", "get folder", "get extension", "get basename", "get side", "get setof", "getID", "getIDStock"}
  T14 = typedef "nameformattingitem.ctl" = enum16{"name", "nameL", "units", "prec"}
  T15 = typedef "cursor action.ctl" = enum16{"range", "read", "write", "check", "zoom out", "smart zoom out", "zoom to aspect ratio 1", "zoom to win", "zoom out 20%", "zoom in 20%", "-empty", "smart zoom out&aspect", "move range left 20%", "move range right 20%", "move range up 20%", "move range down 20%", "zoom to X win", "zoom to Y win", "zoom out X", "zoom out Y", "zoom in X", "zoom in Y", "check plot scale", "set plot color", "set Xlabel", "set Ylabel", "set cursor color", "setlength", "empty", "hide plot", "unhide plot", "checklngth", "extend +1 if short", "extend +n if short"}
  T16 = cluster{"keys":T1[], "regexps":string[], "labels":string[]}
  T17 = typedef "cursor window action.ctl" = enum16{"balance", "h. offset change", "cursor moves", "change center", "change window", "init", "check", "reset", "set y to middle", "idle", "-write all Y", "-write left.X", "-write center.X", "-write right.X", "-write all X", "-change center", "-change window", "-change skew", "-read cursor 2", "-read cursor 1", "-read cursor 0", "-read all cursors", "-reset", "-read plot scale", "-set y to middle", "-Q: center.Y is visible", "-Q: window is visible", "-parse center.Y", "-right left from center", "-left move", "-right move", "-set center.Y", "-empty", "-set cursors to default", "-check", "-write center.Y", "-copy cursor 1", "-copy cursor 0", "-copy cursor 2", "move right", "move left", "shrink", "broaden", "skew up", "skew down", "-write plot scale", "zoom X", "change cen&win", "zoom to all data", "color--red", "color--green", "color--yellow", "read", "zoom out", "zoom in", "slide right", "slide left", "set range aspect ratio to 1", "move to window range", "--move to window range"}
  T18 = typedef "mathematica string map action.ctl" = enum16{"create string", "calc m1m2m3", "parse string"}
  T19 = typedef "3-lorentzian-heat-response action.ctl" = enum16{"calc R", "create string", "calc m1m2m3", "dζ", "dT1", "dτS", "dτN", "dτC", "d-all", "dκ0", "T(K)", "m1", "m2", "m3", "parse string", "θ (deg)", "B (T)", "onlygrads", "newton", "create emty string", "simple2nd", "calc R2", "ScalarProd", "ScalarProd-diff", "nothing", "ScalarProd-eta", "tolog", "ignore", "three2nd", "eta-errors"}
  T20 = typedef "publisher action.ctl" = enum16{"set", "get", "init", "check"}
  T21 = typedef "nanocal -- gradient descent-- data.ctl" = cluster{"dz/dω  (sec/rad)":cdb[], "z ":cdb[], "ω (rad/sec)":dbl[]}
  T22 = typedef "nanocal -- gradient descent -- action.ctl" = enum16{"init", "step", "peek"}
  T23 = typedef "cursor sate.ctl" = enum16{"normal", "alert", "fuzzy", "interesting", "boring", "colored"}
  T24 = typedef "agregator -- action.ctl" = enum16{"append", "interpolate", "empty!", "force", "init", "scale", "read last"}
  T25 = typedef "LVMapReplaceAction.ctl" = enum32{"Modify Entry only if found", "Add or Modify Entry", "Delete Entry"}
  T26 = typedef "nanocal -- defaut parameter manager action-- V1.ctl" = enum16{"get logarithmic interp", "update", "get linear interp"}
  T27 = typedef "nanocal -- plotstring file action.ctl" = enum16{"generate plotstring file", "generate plotstring thing", ""}
  T28 = typedef "file -- read-write control.ctl" = enum16{"read", "write all", "append one line"}
  T29 = typedef "array -- freq-voltage transformations action.ctl" = enum16{"as is", "add -ω", "sort ω", "2 x ω", "R-phase(deg) to Re-Im", "select ω>0", "labview file str", "select |ω|<max", "apply RC transform", "subtract background"}
  T30 = typedef "nanocal_raw_file_manage_action_V1.ctl" = enum16{"read S side", "read R side", "read meta", "read_names"}
  T31 = typedef "KM_file -- read-write control.ctl" = enum16{"read", "write all", "append one line"}
  T32 = typedef "array action.ctl" = enum16{"generate range", "generate log range"}
  T33 = typedef "LVRangeTypeDef.ctl" = cluster{"Minimum":dbl, "Maximum":dbl, "Increment":dbl, "Minor Increment":dbl, "Start":dbl}
  T34 = typedef "interpolation state - real.ctl" = cluster{"Array ":dbl[], "actual size":i32, "requested size":i32}
  T35 = typedef "2Dwindow.ctl" = cluster{"window y":dbl, "center x":dbl, "center y":dbl, "window x":dbl}
